vi "Cal ColNum(SubVI).vi"(9 "EOL":bool, 10 "DV":bool, 11 "PreColNum":i16) -> (3 "CurColNum":i16)   [LabVIEW 2016]
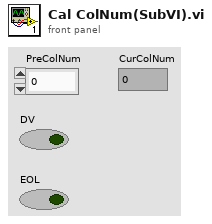
[diagram p1: front panel]
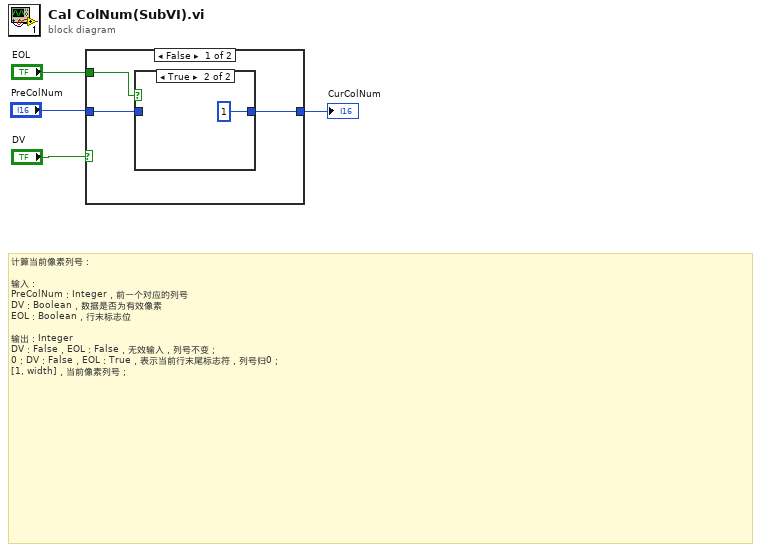
[diagram p0: block diagram]
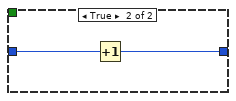
[diagram p3: hidden frame]
diagram:
  # "计算当前像素列号：\n\n输入：\nPreColNum：Integer，前一个对应的列号\nDV：Boolean，数据是否为有效像素\nEOL：Boolean，行末标志位\n\n输出：Integer\nDV：False，EOL：False，无效输入，列号不变；\n0：DV：False，EOL：True，表示当前行末尾标志符，列号归0；\n[1, width]，当前像素列号；"
  n1 = case shown="False" "DV" {
    tunnel: "EOL" -> [w7 _]
    tunnel: [w6 w11] -> w4
    tunnel: "PreColNum" -> [w5 w10]
    frame False {
      n2 = case shown="True" w7 {
        tunnel: [w8 i16 1] -> w6
        tunnel: w5 -> [w8 _]
        frame False {
        }
        frame True {
        }
      }
    }
    frame True {
      n3 = Increment(x=w10) -> (x+1=w11:i16)
    }
  }
  "CurColNum" <- w4
